vi "New Terminate Event.vi"(11 "error in (no error)":errorcluster) -> (4 "Exit Event Ref":T1, 15 "error out":errorcluster)   [LabVIEW 2015, in "TLB` Springboard.lvlib" / "TLB`_Dependencies.lvlib"]
doc: "TLB Prime - Application Template 1.3.0.24\nNorm Kirchner, NI Systems Engineering - NI\nCopyright (c) 2014, NI"
uses:
  TLB`_Dependencies.lvlib
  Exit Event Ref.ctl
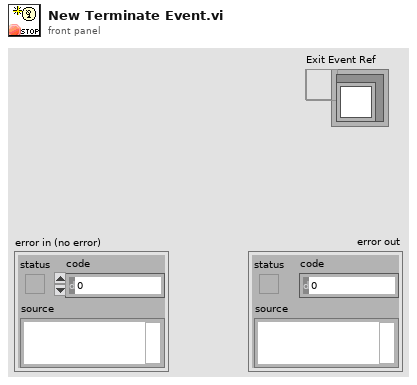
[diagram p1: front panel]
types:
  T1 = typedef "TLB` Springboard.lvlib/TLB`_Dependencies.lvlib/Exit Event Ref.ctl" = refnum<user-event>
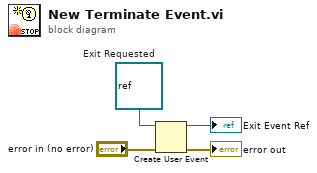
[diagram p0: block diagram]
diagram:
  w4 = refnum<class> refnum  # Exit Requested
  n1 = Create User Event(user event datatype=w4, error in="error in (no error)") -> (user event=→"Exit Event Ref":refnum<user-event>, error out=→"error out":errorcluster)
